vi "U32.vi"(4 "Value":u32) -> (1 "Constant":refnum<class "Const_U32.lvclass">)   [LabVIEW 2021, in "Const_U32.lvclass"]
uses:
  Const_U32.lvclass
  Const_U32.lvclass/Const_U32.ctl
  Properties/Write Value.vi
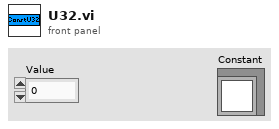
[diagram p1: front panel]
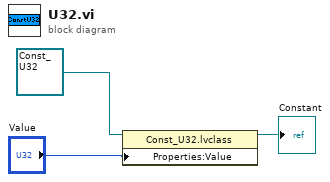
[diagram p0: block diagram]
diagram:
  n1 = property class="Const_U32.lvclass"(reference=refnum<class "Const_U32.lvclass"> refnum ("Constants.lvlib:Numeric.lvclass"), "Properties:Value"="Value") -> (reference out=→"Constant":refnum<class "Const_U32.lvclass">)  [unwired: 1 in, 1 out]
